vi "Channel ctrl disabled synergy.vi"(8 "error in (no error)":errorcluster, 9 "Behaviour":T1, 10 "Right Channel":refnum<vi>, 11 "Left Channel":refnum<vi>) -> (0 "error out":errorcluster)   [LabVIEW 2017]
uses:
  Typedefs/Channel control synergistic behaviour enum.ctl
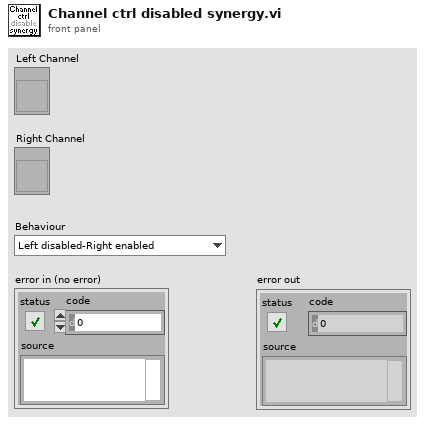
[diagram p1: front panel]
types:
  T1 = typedef "Channel control synergistic behaviour enum.ctl" = enum16{"Left disabled-Right enabled", "Left enabled-Right disabled", "Both enabled"}
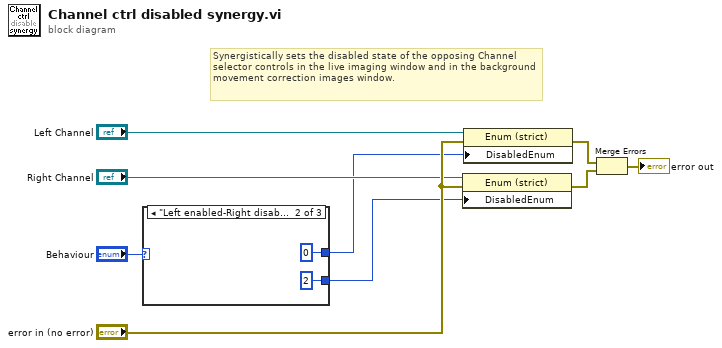
[diagram p0: block diagram]
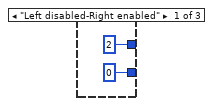
[diagram p2: hidden frame]
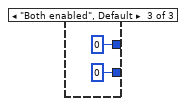
[diagram p3: hidden frame]
diagram:
  # "Synergistically sets the disabled state of the opposing Channel selector controls in the live imaging window and in the background movement correction images window."
  n1 = case shown="\"Left enabled-Right disabled\"" "Behaviour" {
    tunnel: [2 0 0] -> w2
    tunnel: [0 2 0] -> w1
    frame "Left disabled-Right enabled" {
    }
    frame "Left enabled-Right disabled" {
    }
    frame "Both enabled", Default {
    }
  }
  n2 = property on="Property Node" class="Enum (strict)"(reference="Right Channel", error in="error in (no error)", "DisabledEnum"=w1) -> (error out=w9:errorcluster)  [unwired: 1 out]
  n3 = property on="Property Node" class="Enum (strict)"(reference="Left Channel", error in="error in (no error)", "DisabledEnum"=w2) -> (error out=w8:errorcluster)  [unwired: 1 out]
  n4 = Merge Errors(w8, w9) -> (→"error out":errorcluster)
